vi "Scan Module.vi"(0 "#B scans":u32=1300, 1 "Channel":u32(ring)=1 items=["A"=1, "B"=2, "A + B"=3, "C"=4, "A + C"=5, "A + B"=6, "D"=8, "A + D"=9, "B + D"=10, "C + D"=12, "A + B + C + D"=15], 11 "Error In":errorcluster, 12 "Start Acquire?":bool) -> (3 "XY Graph":cluster{"X":dbl, "Y":dbl}[](graph), 4 "Finished?":bool, 6 "Ready for next C-scan?":bool, 8 "Current Position":cluster{"X":dbl, "Y":dbl}, 10 "Current state":T1, 15 "Error Out":errorcluster)   [LabVIEW 2018]
uses:
  Controls/Go Scan Actions.ctl
  Controls/FGV Actions.ctl
  Hardware Mfg/Thorlabs Translation Stages/Controls/Motion Translation Module Control.ctl
  Controls/Set Get Controls.ctl
  Hardware Mfg/Thorlabs Translation Stages/Controls/Translation Stage Cluster.ctl
  Controls/Translation Stage Types.ctl
  Hardware Mfg/AlazarTech SDK/Controls/Alazar Engine Actions.ctl
panel:
  out "Waveform Chart":dbl(graph)
  in  "No Slice?":bool
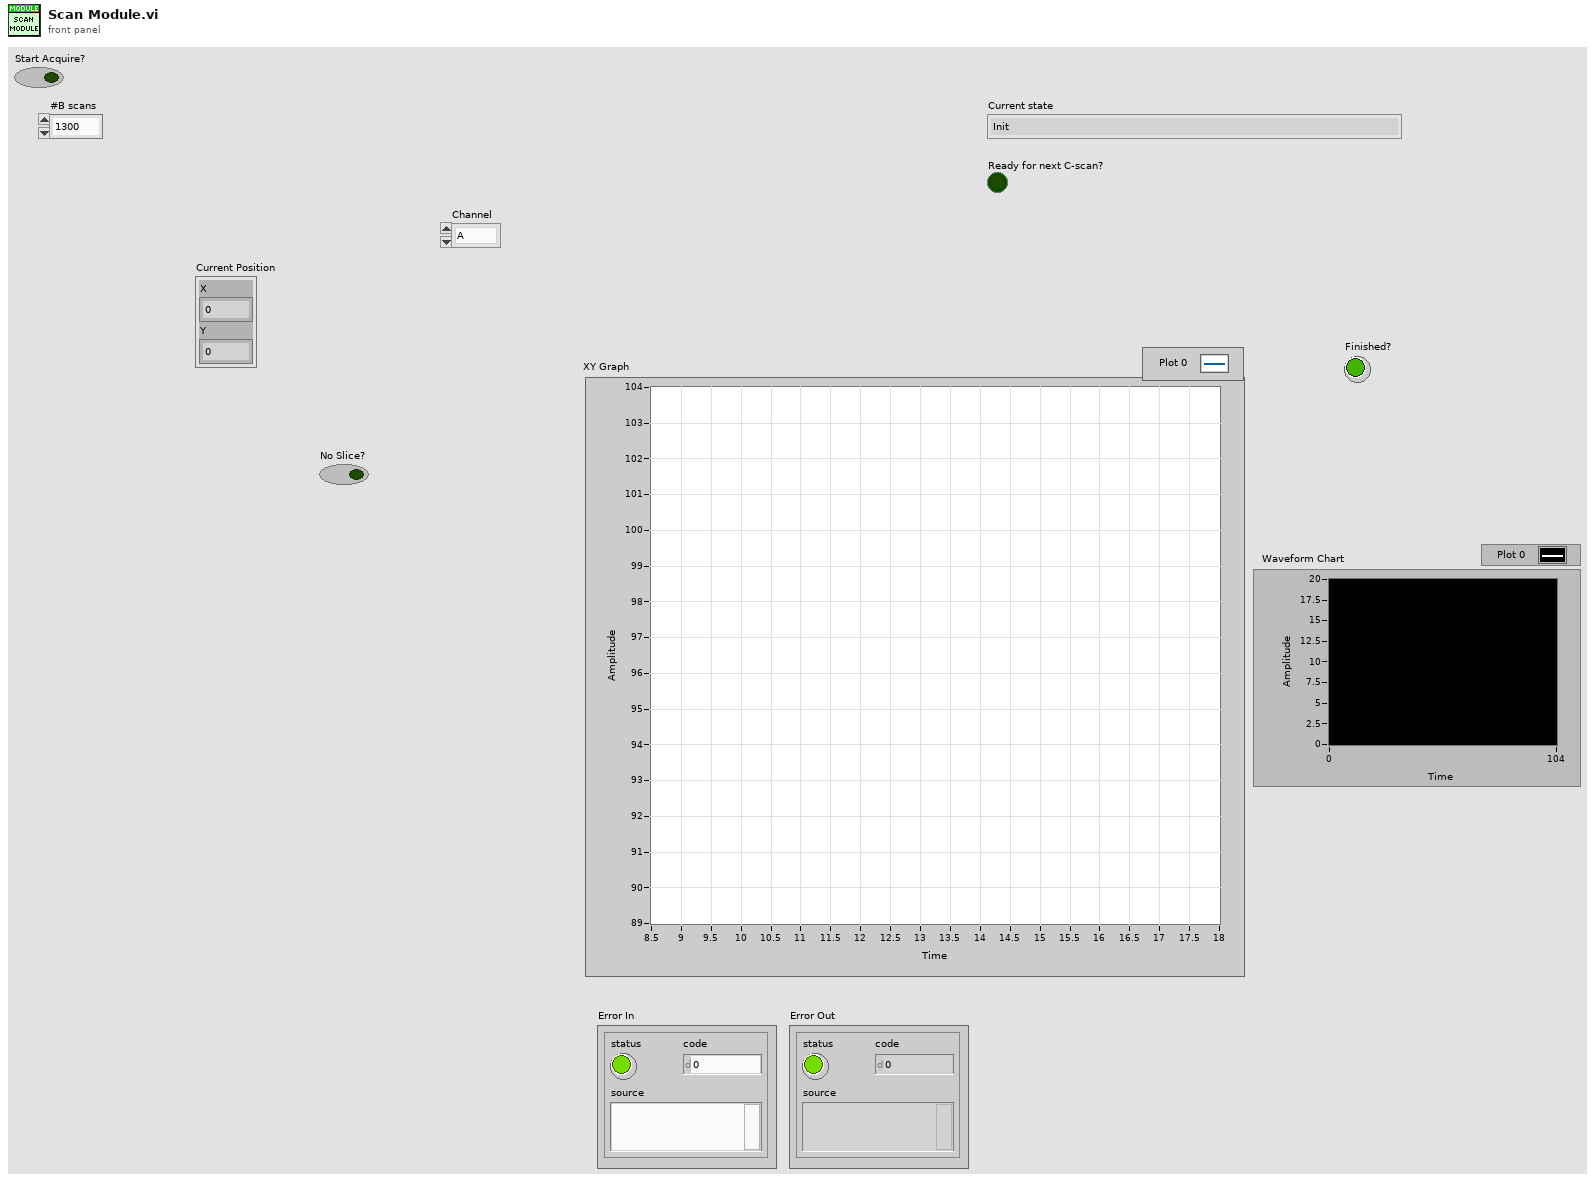
[diagram p1: front panel]
types:
  T1 = typedef "Go Scan Actions.ctl" = enum16{"Init", "Ready for acquire", "Init Scan Head", "Init Table Stage", "Init Vibratome", "Generate Mosaic", "Export info", "Go Image Home", "Go Mosaic", "Acquire Image", "Go Vibratome", "Slice", "Finished"}
  T2 = typedef "FGV Actions.ctl" = enum16{"Init", "Set", "Get", "Clear"}
  T3 = typedef "Translation Stage Cluster.ctl" = cluster{"Position":dbl, "Is.Enabled?":bool, "Is.Connected?":bool, "Device SN":string, "AccelerationMaximum":dbl, "VelocityMaximum":dbl, "Acceleration":dbl, "Velocity":dbl, "waitTimeout (ms)":i32, "Model":T4, "Is.Homed?":bool}
  T4 = typedef "Translation Stage Types.ctl" = enum16{"None", "Thorlabs LTS", "Thorlabs MLJ"}
  T5 = typedef "Set Get Controls.ctl" = enum16{"Set", "Get"}
  T6 = typedef "Motion Translation Module Control.ctl" = enum16{"Init", "Home", "Status", "Velocity/Accel", "Position", "Jog", "Stop", "Uninit", "Enable", "Disable"}
  T7 = enum16{"Configure channels", "Write Scan Pattern", "Start Galvo Task", "Is Task Done?", "Stop Galvo", "Uninit", "Init: Calc scan pattern"}
  T8 = typedef "Alazar Engine Actions.ctl" = enum16{"Init", "Config Clock", "Config Ch", "Config Trig", "Config Non-FFT Acq.", "Non-FFT Acquire", "Load background from Non-FFT buffer", "enable background subtrac", "disable background subtrac", "load background from file", "load background from elsewhere", "start acquire", "background subtraction", "Config Acq.", "Acquire", "UnInit"}
  T9 = typedef "Hardware control.ctl" = enum16{"PSOCT", "Thorlabs OCT"}
  T10 = typedef "ScanType.ctl" = enum16{"Single Frame", "Continuous Frame", "ROI Line", "Vibratome", "Mosaic", "Mosaic + Slice"}
  T11 = typedef "System Parameters.ctl" = cluster{"Optical Parameters":T12, "Vibratome":T13, "Table Stages":T14, "Imaging Parameter":T15, "Galvo HW Parameters":cluster{"Analog Out Channel":tag, "Min Voltage":dbl, "Max Voltage":dbl, "Pixel Clock Source":tag, "Sample Rate":dbl, "Line Clock Out Ch":tag}, "Alazar parameters":T17, "Mosaic Paramter":cluster{"X Axis":cluster{"Start [mm]":dbl, "Steps [pts]":u16, "End [mm]":dbl}, "Y Axis":cluster{"Start [mm]":dbl, "Steps [pts]":u16, "End [mm]":dbl}, "Scan Pattern":enum16{"Uni-directional", "Bi-Directional", "Spiral Out", "Spiral In"}, "Overlap Options":cluster{"Overlap Type":enum16{"No Overlap", "X Only", "Y Only", "X and Y"}, "Percent Overlap":u8, "Justify":enum16{"Start", "Center", "End"}}}}
  T12 = typedef "Optical Parameters.ctl" = cluster{"Obj. Focal Length [mm]":dbl, "Scan Lens EFL[mm]":dbl, "Tube Lens EFL[mm]":dbl, "Galvo V Range (+/-)":dbl, "Galvo Max Half Angle [Deg]":dbl, "Max Galvo Range[%]":dbl}
  T13 = typedef "Vibratome Parameters.ctl" = cluster{"Z Bottom [mm]":dbl, "Pre Cut Dwell [s]":dbl, "Blade Frequency [RPM]":u16, "Slice Speed [mm/s]":dbl, "Post Cut Dwell [s]":dbl, "Ramp Time [s]":dbl, "Start X [mm]":dbl, "Start Y [mm]":dbl, "Slice Length [mm]":dbl, "Slice Axis":enum16{"X Axis", "Y Axis", "Z Axis"}, "Controller VISA Ref":refnum<visa-resource-name>}
  T14 = typedef "Translation Stage Parameters.ctl" = cluster{"X Stage":T3, "Y Stage":T3, "Z Stage":T3}
  T15 = typedef "Imaging Parameters.ctl" = cluster{"Raster Scan Direction":T16, "Pixel Dwell Time [Clock Cycles]":u16, "Flyback Time [Clock Cycles]":u16, "XY Center [um]":cluster{"X":dbl, "Y":dbl}, "Pixel Step Size [um]":dbl, "XY Image Size":enum16{"32 x 32", "64 x 64", "128 x 128", "256 x 256", "512 x 512", "1024 x 1024", "2048 x 2048"}, "Custom":bool, "Custom Size":cluster{"X":u16, "Y":u16}, "Line Averages":u8}
  T16 = typedef "Scan Direction.ctl" = enum16{"Uni Directional", "Bi Directional", "None"}
  T17 = typedef "Alazar parameters.ctl" = cluster{"Trigger Settings":cluster{"General Trigger Settings":T18, "Trigger Engine 1":T19, "Trigger Engine 2":T19}, "Capture Clock":T20, "Device ID":T21, "Ch A Input Control":T22, "Ch B Input Control":T22, "Acq Settings":T23}
  T18 = typedef "General Trigger Settings.ctl" = cluster{"Trigger Operation":u32, "Coupling ID":u32, "Range ID":u32, "Delay":u32, "Timeout Ticks":u32, "Mode":u32, "Parameter":u32}
  T19 = typedef "Trigger Engine Controls.ctl" = cluster{"Trigger Engine":u32, "Source":u32, "Slope":u32, "Level":u32}
  T20 = typedef "Clock Controls.ctl" = cluster{"Sample Rate":u32, "Decimation":u32, "Source":u32, "Edge":u32}
  T21 = typedef "Alazar Device ID.ctl" = cluster{"System ID":u32, "Board ID":u32}
  T22 = typedef "Channel Input Controls.ctl" = cluster{"Channel":u8, "Coupling":u32, "Range":u32, "Impedance":u32}
  T23 = typedef "Alazar Acquisition Settings.ctl" = cluster{"Window Type":u32, "Record Length":u32, "Footer":u32, "Offset":u32, "Records Per Buffer":u32, "Samples per record":u32, "Records Count (Records/Acq)":u32, "Output Format":u32}
  T24 = cluster{"X Axis":cluster{"Start [mm]":dbl, "Steps [pts]":u16, "End [mm]":dbl}, "Y Axis":cluster{"Start [mm]":dbl, "Steps [pts]":u16, "End [mm]":dbl}, "Scan Pattern":enum16{"Uni-directional", "Bi-Directional", "Spiral Out", "Spiral In"}, "Overlap Options":cluster{"Overlap Type":enum16{"No Overlap", "X Only", "Y Only", "X and Y"}, "Percent Overlap":u8, "Justify":enum16{"Start", "Center", "End"}}}
  T25 = cluster{"Start [mm]":dbl, "Steps [pts]":u16, "End [mm]":dbl}
  T26 = cluster{"Overlap Type":enum16{"No Overlap", "X Only", "Y Only", "X and Y"}, "Percent Overlap":u8, "Justify":enum16{"Start", "Center", "End"}}
  T27 = enum16{"Uni-directional", "Bi-Directional", "Spiral Out", "Spiral In"}
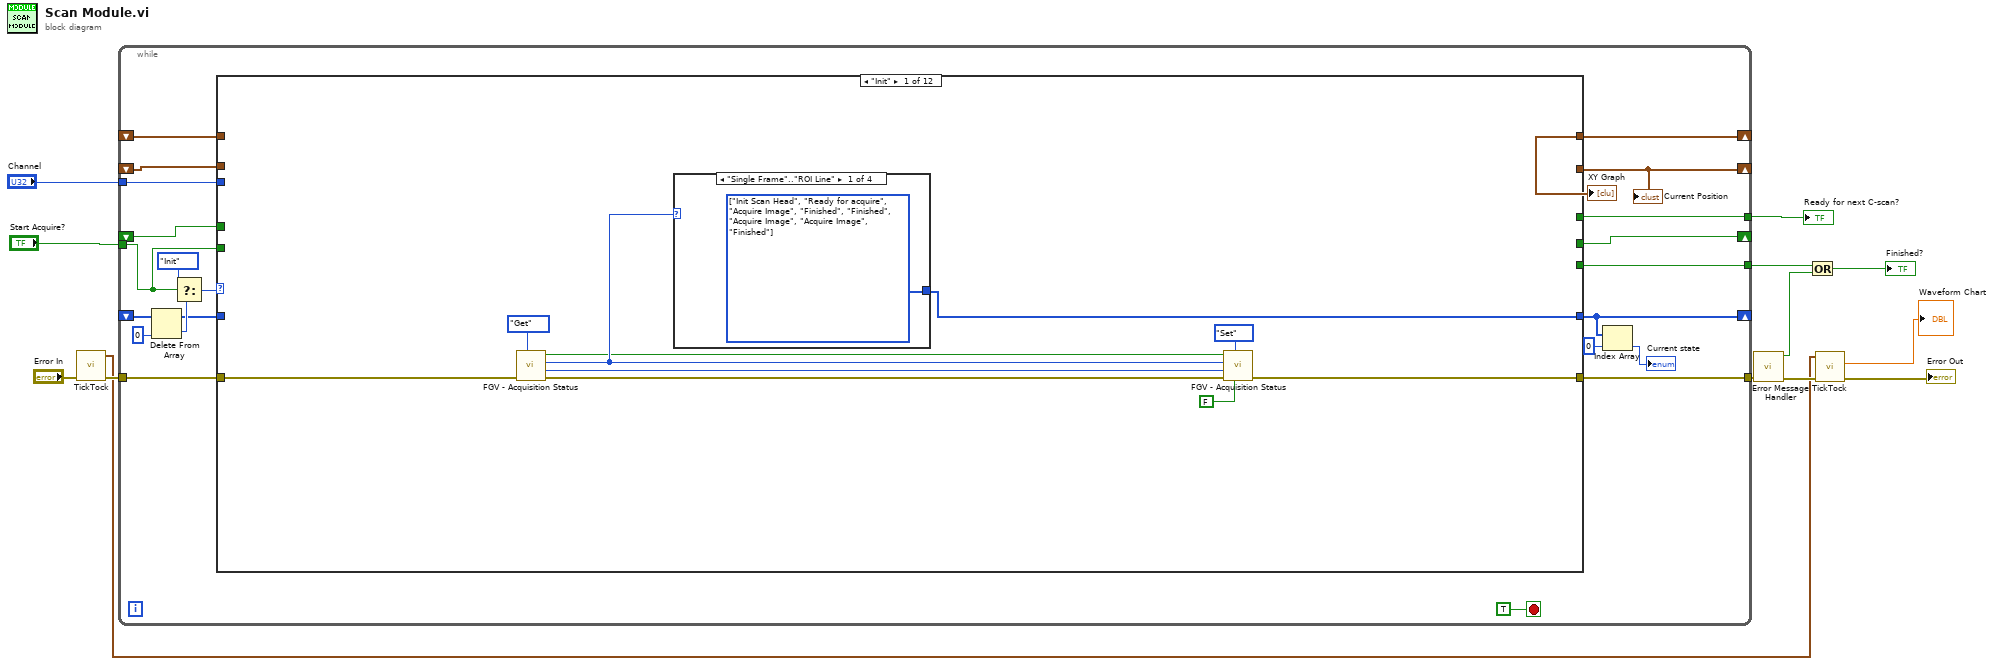
[diagram p0: block diagram]
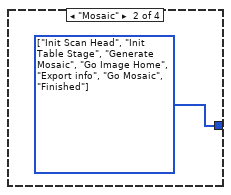
[diagram p2: hidden frame]
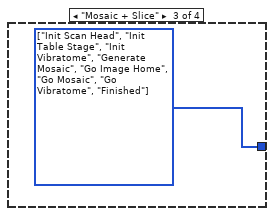
[diagram p3: hidden frame]
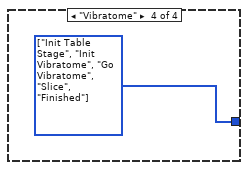
[diagram p4: hidden frame]
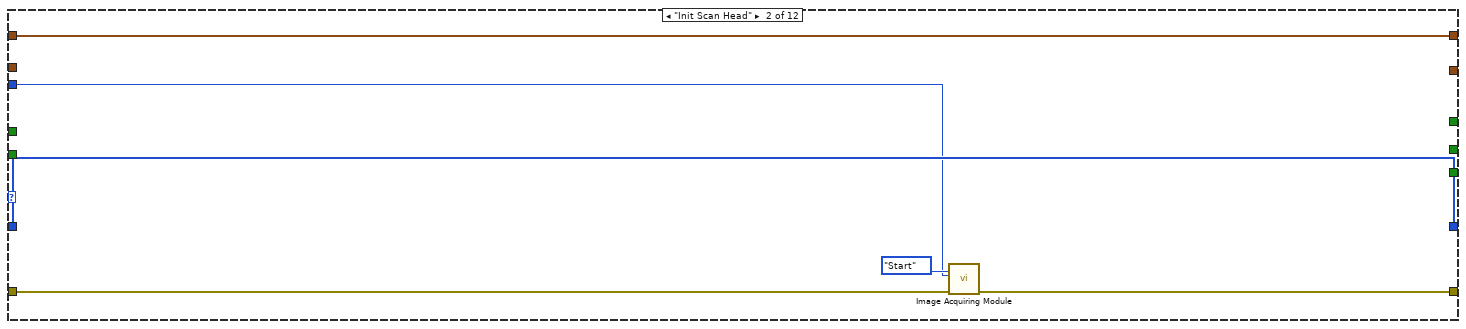
[diagram p5: hidden frame]
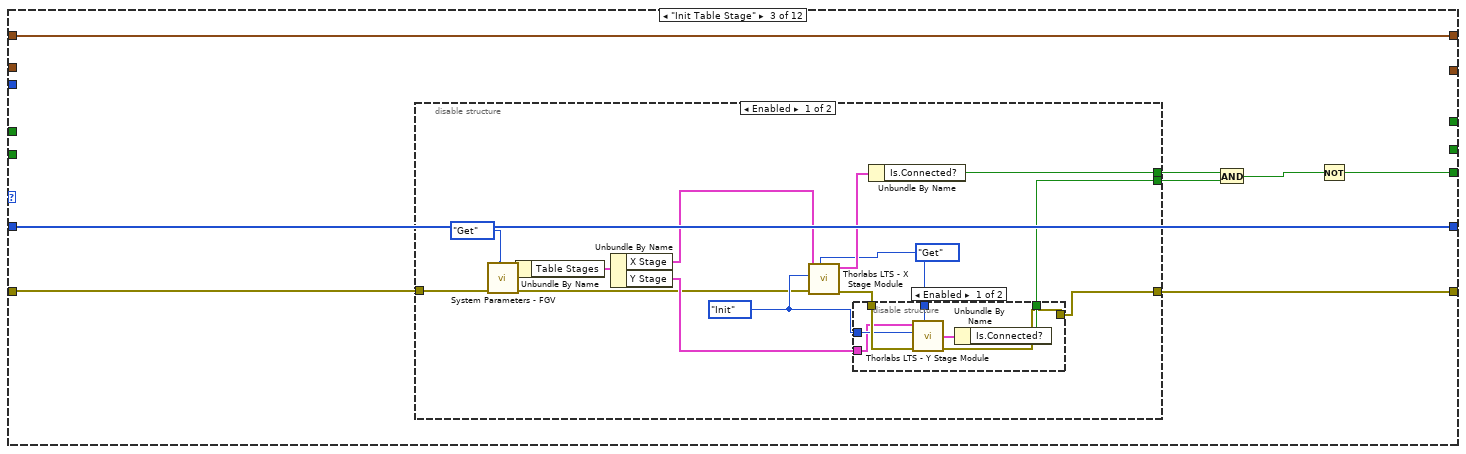
[diagram p6: hidden frame]
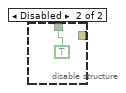
[diagram p7: hidden frame]
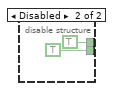
[diagram p8: hidden frame]
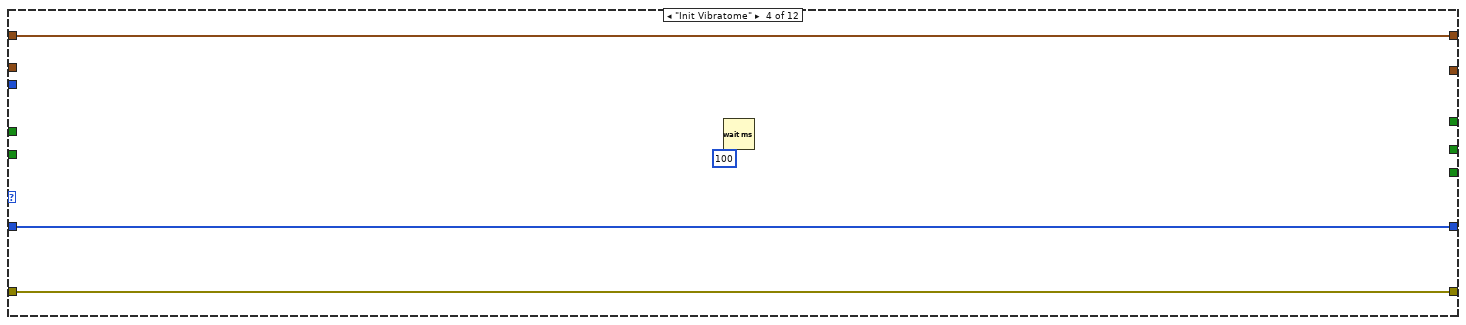
[diagram p9: hidden frame]
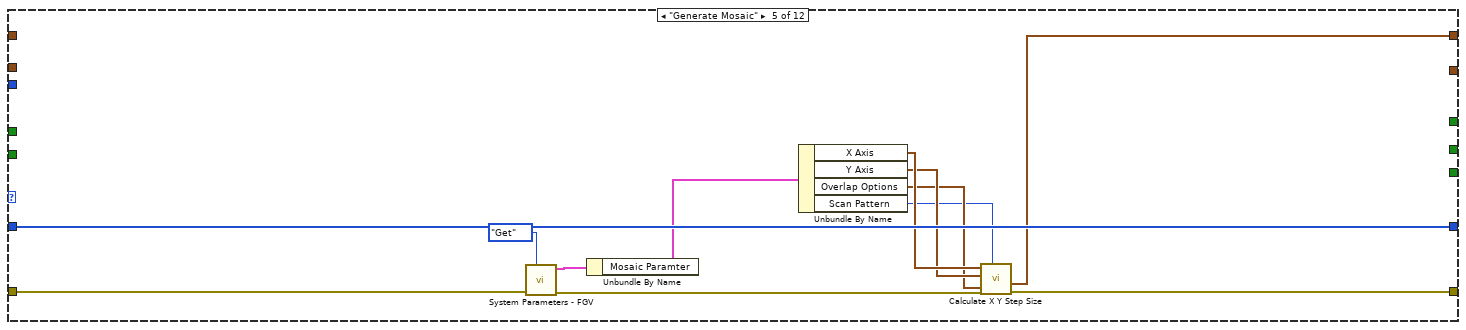
[diagram p10: hidden frame]
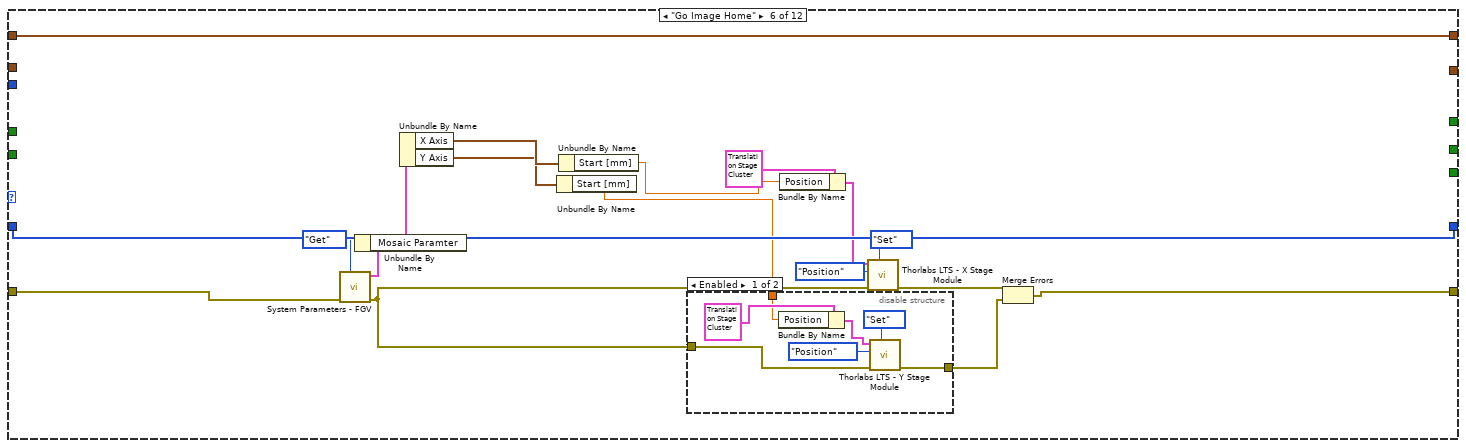
[diagram p11: hidden frame]
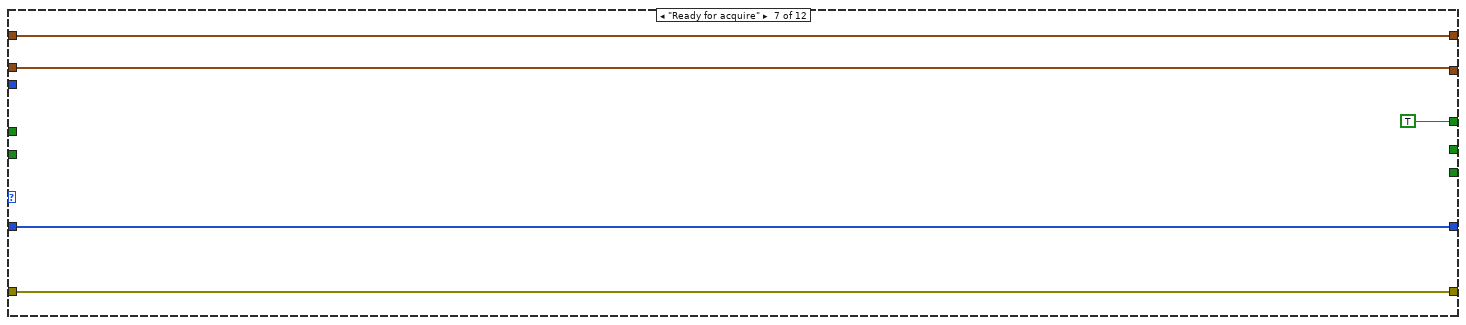
[diagram p13: hidden frame]
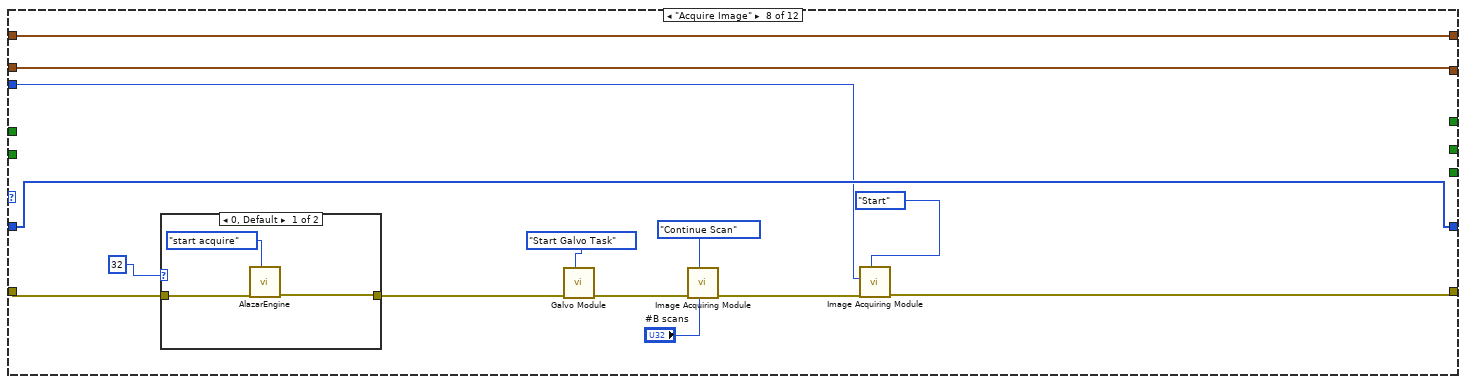
[diagram p14: hidden frame]
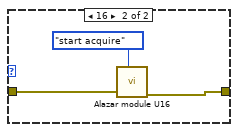
[diagram p15: hidden frame]
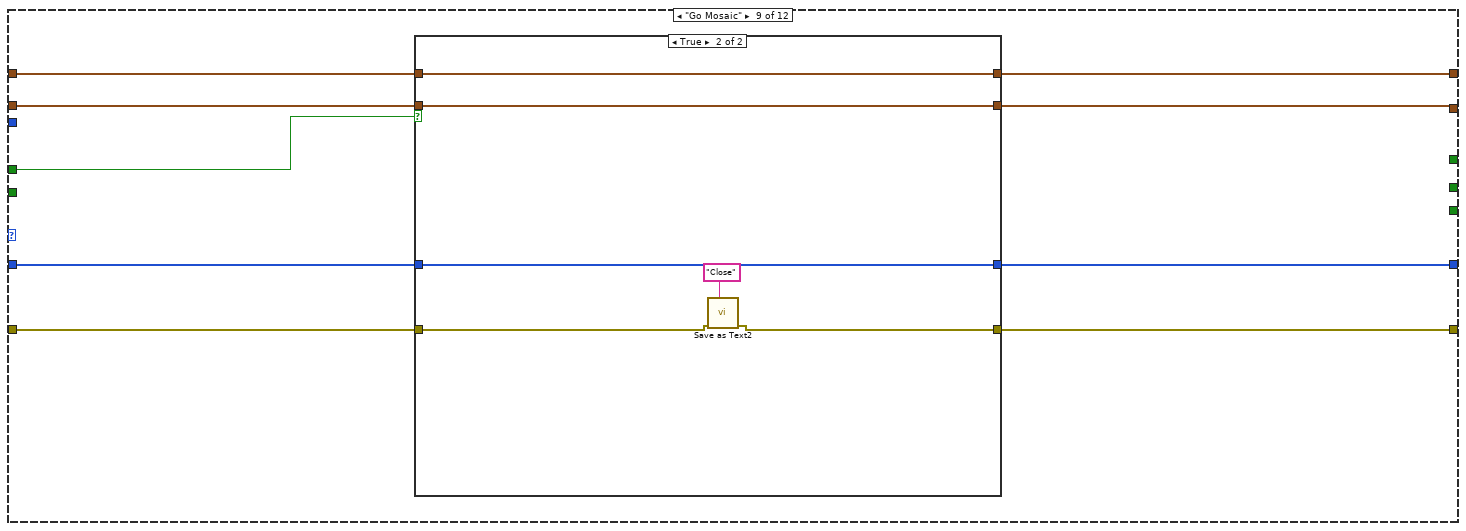
[diagram p16: hidden frame]
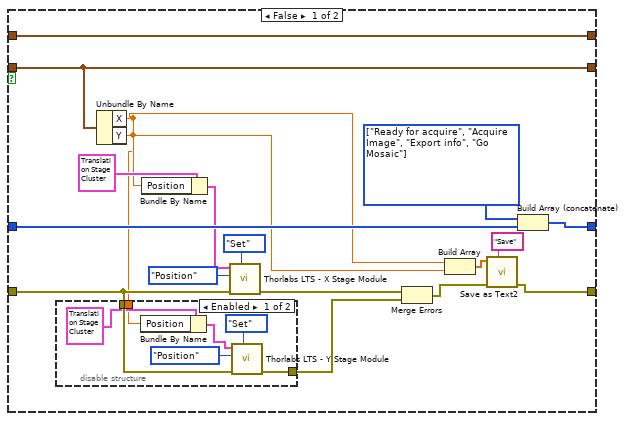
[diagram p17: hidden frame]
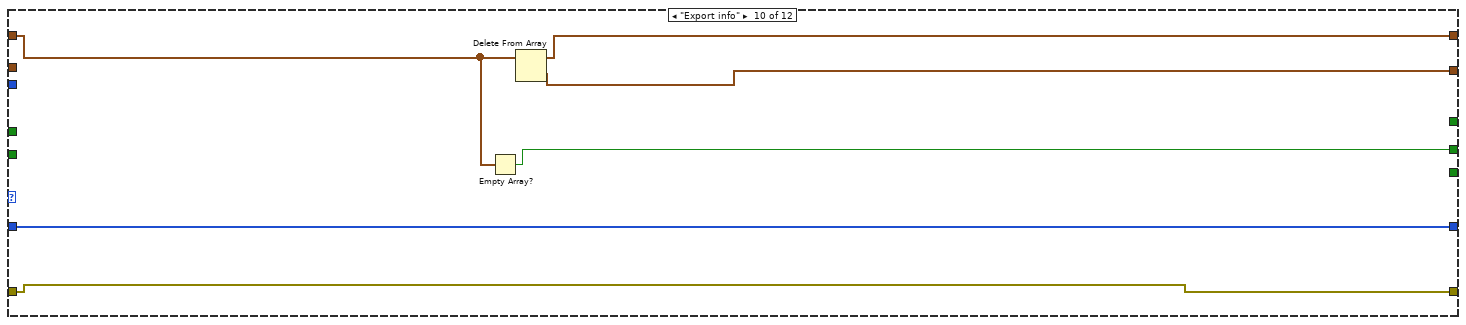
[diagram p19: hidden frame]
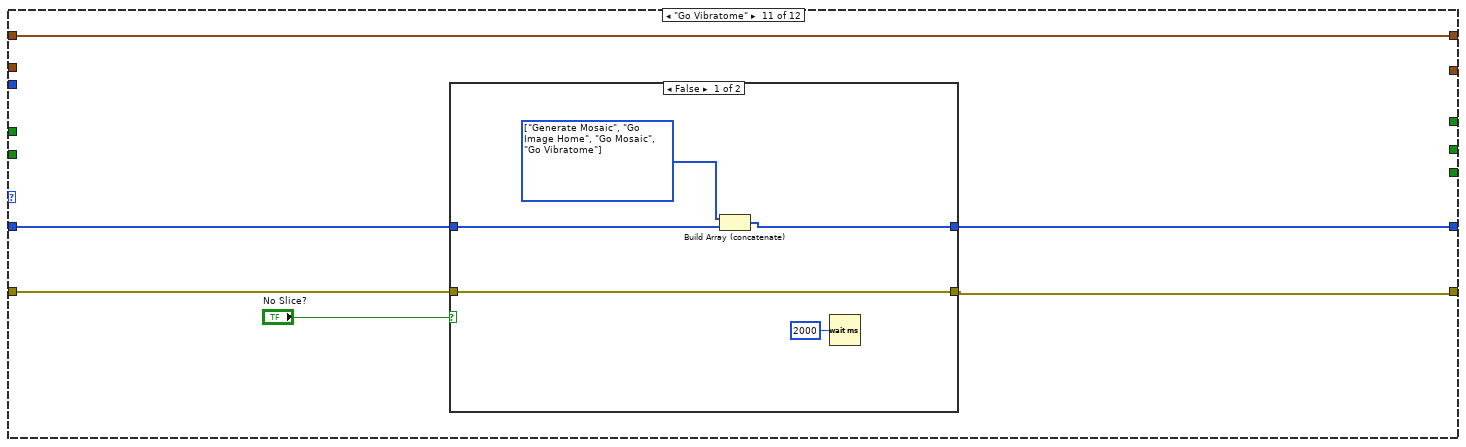
[diagram p20: hidden frame]
diagram:
  n1 = call "TickTock.vi"("Error In"="Error In") -> ("Error Out"=w7:errorcluster, "Current Time (Out)"=w5:timestamp)  [unwired: 8 in, 1 out]
  n2 = while {
    shift-right: [w16] -> _
    shift-left: _ -> [w33]
    tunnel: "Start Acquire?" -> [w23]
    shift-right: [w29] -> _
    shift-left: _ -> [w30]
    tunnel: [w28] -> w13
    tunnel: w7 -> [w26]
    tunnel: [w25] -> w12
    tunnel: [w22] -> w2
    tunnel: "Channel" -> [w21]
    shift-right: [w14] -> _
    shift-left: _ -> [w18]
    shift-right: [w20] -> _
    shift-left: _ -> [w19]
    stop <- TRUE stop-if-true
    n3 = Delete From Array(array=w33, index=0) -> (deleted portion=w32:T1, array with subset deleted=w31:T1[])  [unwired: 1 in]
    n4 = Select(t=Go_Scan_Actions."Init", s=w23, f=w32) -> (s? t:f=w24:T1)
    n5 = case shown="\"Init\"" w24 {
      tunnel: [w43 w54 w62 w90 w103 w121 w130 w146 w157 w196 w200 _] -> w16
      tunnel: w31 -> [_ w54 w62 w90 w103 w121 w130 w146 w160 w196 w203 _]
      tunnel: [_ w55 w63 w91 w102 w120 w132 w147 w162 w199 w205 _] -> w29
      tunnel: w30 -> [_ w55 w63 w91 _ w120 w132 w147 w161 w198 w205 _]
      tunnel: [_ _ w60 _ _ _ _ _ _ _ _ TRUE] -> w28
      tunnel: w26 -> [w44 w50 w57 w88 w93 w106 w133 w142 w159 w194 w202 w222]
      tunnel: [w41 w52 w56 w88 w92 w104 w133 w138 w158 w194 w201 w214] -> w25
      tunnel: w23 -> [_ _ _ _ _ _ _ _ _ _ _ _]
      tunnel: [_ _ _ _ _ _ TRUE _ _ _ _ _] -> w22
      tunnel: w21 -> [_ w51 _ _ _ _ _ w139 _ _ _ _]
      tunnel: [_ _ _ _ _ _ w129 w134 w154 w195 _ _] -> w14
      tunnel: [_ _ _ _ _ _ _ _ _ w197 _ _] -> w20
      tunnel: w19 -> [_ _ _ _ _ _ _ _ w156 _ _ _]
      tunnel: w18 -> [_ _ _ _ _ _ w129 w134 w155 _ _ _]
      frame "Init" {
        n6 = call "FGV - Acquisition Status.vi"("Actions"=FGV_Actions."Get", "Error In"=w44) -> ("Error Out"=w42:errorcluster, "Hardware out"=w39:T9, "Scan Type [Out]"=w38:T10, "Level Status Out"=w37:bool)  [unwired: 5 in, 1 out]
        n7 = case shown="\"Single Frame\"..\"ROI Line\"" w38 {
          tunnel: [w46 w47 w48 w49] -> w43
          frame "Single Frame".."ROI Line" {
            w46 = T1[] [enum."Init Scan Head", enum."Ready for acquire", enum."Acquire Image", enum."Finished", enum."Finished", enum."Acquire Image", enum."Acquire Image", enum."Finished"] items=["Init", "Ready for acquire", "Init Scan Head", "Init Table Stage", "Init Vibratome", "Generate Mosaic", "Export info", "Go Image Home", "Go Mosaic", "Acquire Image", "Go Vibratome", "Slice", "Finished"]
          }
          frame "Mosaic" {
            w47 = T1[] [enum."Init Scan Head", enum."Init Table Stage", enum."Generate Mosaic", enum."Go Image Home", enum."Export info", enum."Go Mosaic", enum."Finished"] items=["Init", "Ready for acquire", "Init Scan Head", "Init Table Stage", "Init Vibratome", "Generate Mosaic", "Export info", "Go Image Home", "Go Mosaic", "Acquire Image", "Go Vibratome", "Slice", "Finished"]
          }
          frame "Mosaic + Slice" {
            w48 = T1[] [enum."Init Scan Head", enum."Init Table Stage", enum."Init Vibratome", enum."Generate Mosaic", enum."Go Image Home", enum."Go Mosaic", enum."Go Vibratome", enum."Finished"] items=["Init", "Ready for acquire", "Init Scan Head", "Init Table Stage", "Init Vibratome", "Generate Mosaic", "Export info", "Go Image Home", "Go Mosaic", "Acquire Image", "Go Vibratome", "Slice", "Finished"]
          }
          frame "Vibratome" {
            w49 = T1[] [enum."Init Table Stage", enum."Init Vibratome", enum."Go Vibratome", enum."Slice", enum."Finished"] items=["Init", "Ready for acquire", "Init Scan Head", "Init Table Stage", "Init Vibratome", "Generate Mosaic", "Export info", "Go Image Home", "Go Mosaic", "Acquire Image", "Go Vibratome", "Slice", "Finished"]
          }
        }
        n8 = call "FGV - Acquisition Status.vi"("Edge Status In"=FALSE, "Actions"=FGV_Actions."Set", "Error In"=w42, "Hardware in"=w39, "Scan Type [In]"=w38, "Level Status In"=w37) -> ("Error Out"=w41:errorcluster)  [unwired: 1 in, 4 out]
      }
      frame "Init Scan Head" {
        n9 = call "Image Acquiring Module.vi"("Scan Status in"=enum16{"Start", "Continue Scan", "Finish Scan"}."Start", "Error in"=w50, "Channel"=w51) -> ("Error Out"=w52:errorcluster)  [unwired: 8 in]
      }
      frame "Init Table Stage" {
        n10 = disable-structure shown="Enabled" {
          disable-tunnel: [w75 TRUE ("Is.Connected?")] -> w61
          disable-tunnel: [w73 TRUE ("Is.Connected?")] -> w58
          disable-tunnel: w57 -> [w66 _]
          disable-tunnel: [w64 _] -> w56
          frame Enabled {
            w72 = Set_Get_Controls."Get" ("Set/Get")
            w74 = Motion_Translation_Module_Control."Init" ("Action")
            n11 = call "System Parameters - FGV.vi"("Actions"=FGV_Actions."Get", "Error In"=w66) -> ("Error Out"=w65:errorcluster, "System Parameters"=w70:T11)  [unwired: 8 in]
            n12 = Unbundle By Name(w70) -> ("Table Stages"=w69:T14)
            n13 = Unbundle By Name(w69) -> ("X Stage"=w68:T3, "Y Stage"=w67:T3)
            n14 = call "Thorlabs LTS - X Stage Module.vi"("Set/Get"=w72, "Error In"=w65, "Action"=w74, "Cluster In"=w68) -> ("Error Out"=w77:errorcluster, "Cluster Out"=w76:T3)  [unwired: 6 in]
            n15 = disable-structure shown="Enabled" {
              disable-tunnel: w77 -> [w84 _]
              disable-tunnel: w74 -> [w83 _]
              disable-tunnel: [w81 TRUE] -> w73
              disable-tunnel: w72 -> [w80 _]
              disable-tunnel: w67 -> [w79 _]
              disable-tunnel: [w78 _] -> w64
              frame Enabled {
                n16 = call "Thorlabs LTS - Y Stage Module.vi"("Set/Get"=w80, "Error In"=w84, "Action"=w83, "Cluster In"=w79) -> ("Error Out"=w78:errorcluster, "Cluster Out"=w82:T3)  [unwired: 6 in]
                n17 = Unbundle By Name(w82) -> ("Is.Connected?"=w81:bool)
              }
              frame Disabled {
              }
            }
            n18 = Unbundle By Name(w76) -> ("Is.Connected?"=w75:bool)
          }
          frame Disabled {
          }
        }
        n19 = And(x=w61, y=w58) -> (x .and. y?=w59:bool)
        n20 = Not(x=w59) -> (.not. x?=w60:bool)
      }
      frame "Init Vibratome" {
        n21 = Wait (ms)(milliseconds to wait=u32 100) -> ()  [unwired: 1 out]
      }
      frame "Generate Mosaic" {
        n22 = call "System Parameters - FGV.vi"("Actions"=FGV_Actions."Get", "Error In"=w93) -> ("Error Out"=w97:errorcluster, "System Parameters"=w95:T11)  [unwired: 8 in]
        n23 = Unbundle By Name(w95) -> ("Mosaic Paramter"=w94:T24)
        n24 = Unbundle By Name(w94) -> ("X Axis"=w101:T25, "Y Axis"=w100:T25, "Overlap Options"=w99:T26, "Scan Pattern"=w98:T27)
        n25 = call "Calculate X Y Step Size.vi"("Overlap Options"=w99, "Scan Pattern"=w98, "Error In"=w97, "Y Axis"=w100, "X Axis"=w101) -> ("Error Out"=w92:errorcluster, "Array"=w102:cluster{"X":dbl, "Y":dbl}[])  [unwired: 3 in, 2 out]
      }
      frame "Go Image Home" {
        n26 = call "System Parameters - FGV.vi"("Actions"=FGV_Actions."Get", "Error In"=w106) -> ("Error Out"=w105:errorcluster, "System Parameters"=w112:T11)  [unwired: 8 in]
        n27 = Unbundle By Name(w112) -> ("Mosaic Paramter"=w111:T24)
        n28 = Unbundle By Name(w111) -> ("X Axis"=w110:T25, "Y Axis"=w109:T25)
        n29 = Unbundle By Name(w109) -> ("Start [mm]"=w107:dbl)
        n30 = Unbundle By Name(w110) -> ("Start [mm]"=w108:dbl)
        n31 = disable-structure shown="Enabled" {
          disable-tunnel: [w124 _] -> w114
          disable-tunnel: w107 -> [w123 _]
          disable-tunnel: w105 -> [w122 _]
          frame Enabled {
            n32 = Bundle By Name(cluster=T3 {"Position"=0.0, "Is.Enabled?"=FALSE, "Is.Connected?"=FALSE, "Device SN"="45876539", "AccelerationMaximum"=0.0, "VelocityMaximum"=0.0, "Acceleration"=0.0, "Velocity"=0.0, "waitTimeout (ms)"=10000, "Model"=enum."None", "Is.Homed?"=FALSE} ("Cluster In"), "Position"=w123) -> (w125:T3)
            n33 = call "Thorlabs LTS - Y Stage Module.vi"("Set/Get"=Set_Get_Controls."Set", "Error In"=w122, "Action"=Motion_Translation_Module_Control."Position", "Cluster In"=w125) -> ("Error Out"=w124:errorcluster)  [unwired: 6 in, 1 out]
          }
          frame Disabled {
          }
        }
        n34 = Bundle By Name(cluster=T3 {"Position"=0.0, "Is.Enabled?"=FALSE, "Is.Connected?"=FALSE, "Device SN"="45876539", "AccelerationMaximum"=0.0, "VelocityMaximum"=0.0, "Acceleration"=0.0, "Velocity"=0.0, "waitTimeout (ms)"=10000, "Model"=enum."None", "Is.Homed?"=FALSE} ("Cluster In"), "Position"=w108) -> (w115:T3)
        n35 = call "Thorlabs LTS - X Stage Module.vi"("Set/Get"=Set_Get_Controls."Set", "Error In"=w105, "Action"=Motion_Translation_Module_Control."Position", "Cluster In"=w115) -> ("Error Out"=w118:errorcluster)  [unwired: 6 in, 1 out]
        n36 = Merge Errors(w118, w114) -> (w104:errorcluster)
      }
      frame "Ready for acquire" {
      }
      frame "Acquire Image" {
        n37 = case shown="0, Default" 32 {
          tunnel: w142 -> [w150 w153]
          tunnel: [w149 w152] -> w137
          frame 0, Default {
            n38 = call "AlazarEngine.vi"("Action"=Alazar_Engine_Actions."start acquire", "error in (no error)"=w150) -> ("error out"=w149:errorcluster)  [unwired: 7 in, 2 out]
          }
          frame 16 {
            n39 = call "Alazar module U16.vi"("Action"=Alazar_Engine_Actions."start acquire", "error in (no error)"=w153) -> ("error out"=w152:errorcluster)  [unwired: 7 in, 2 out]
          }
        }
        n40 = call "Galvo Module.vi"("Action"=T7."Start Galvo Task", "error in (no error)"=w137) -> ("error out"=w143:errorcluster)  [unwired: 8 in, 1 out]
        n41 = call "Image Acquiring Module.vi"("#B scans"="#B scans", "Scan Status in"=enum16{"Start", "Continue Scan", "Finish Scan"}."Continue Scan", "Error in"=w143) -> ("Error Out"=w141:errorcluster)  [unwired: 8 in]
        n42 = call "Image Acquiring Module.vi"("Scan Status in"=enum16{"Start", "Continue Scan", "Finish Scan"}."Start", "Error in"=w141, "Channel"=w139) -> ("Error Out"=w138:errorcluster)  [unwired: 8 in]
      }
      frame "Go Mosaic" {
        n43 = case shown="True" w156 {
          tunnel: [w170 w193] -> w162
          tunnel: w161 -> [w170 w193]
          tunnel: w160 -> [w180 w192]
          tunnel: [w179 w192] -> w157
          tunnel: w159 -> [w172 w189]
          tunnel: [w166 w188] -> w158
          tunnel: w155 -> [w163 w191]
          tunnel: [w163 w191] -> w154
          frame False {
            w178 = T1[] [enum."Ready for acquire", enum."Acquire Image", enum."Export info", enum."Go Mosaic"] items=["Init", "Ready for acquire", "Init Scan Head", "Init Table Stage", "Init Vibratome", "Generate Mosaic", "Export info", "Go Image Home", "Go Mosaic", "Acquire Image", "Go Vibratome", "Slice", "Finished"]
            n44 = Unbundle By Name(w163) -> ("X"=w165:dbl, "Y"=w164:dbl)
            n45 = disable-structure shown="Enabled" {
              disable-tunnel: w172 -> [w185 _]
              disable-tunnel: w164 -> [w183 _]
              disable-tunnel: [w181 _] -> w171
              frame Enabled {
                n46 = Bundle By Name(cluster=T3 {"Position"=0.0, "Is.Enabled?"=FALSE, "Is.Connected?"=FALSE, "Device SN"="45876539", "AccelerationMaximum"=0.0, "VelocityMaximum"=0.0, "Acceleration"=0.0, "Velocity"=0.0, "waitTimeout (ms)"=10000, "Model"=enum."None", "Is.Homed?"=FALSE} ("Cluster In"), "Position"=w183) -> (w182:T3)
                n47 = call "Thorlabs LTS - Y Stage Module.vi"("Set/Get"=Set_Get_Controls."Set", "Error In"=w185, "Action"=Motion_Translation_Module_Control."Position", "Cluster In"=w182) -> ("Error Out"=w181:errorcluster)  [unwired: 6 in, 1 out]
              }
              frame Disabled {
              }
            }
            n48 = Bundle By Name(cluster=T3 {"Position"=0.0, "Is.Enabled?"=FALSE, "Is.Connected?"=FALSE, "Device SN"="45876539", "AccelerationMaximum"=0.0, "VelocityMaximum"=0.0, "Acceleration"=0.0, "Velocity"=0.0, "waitTimeout (ms)"=10000, "Model"=enum."None", "Is.Homed?"=FALSE} ("Cluster In"), "Position"=w165) -> (w173:T3)
            n49 = call "Thorlabs LTS - X Stage Module.vi"("Set/Get"=Set_Get_Controls."Set", "Error In"=w172, "Action"=Motion_Translation_Module_Control."Position", "Cluster In"=w173) -> ("Error Out"=w176:errorcluster)  [unwired: 6 in, 1 out]
            n50 = Merge Errors(w176, w171) -> (w167:errorcluster)
            n51 = Build Array(w165, w164) -> (w169:dbl[])
            n52 = call "Save as Text2.vi"("action"="Save", "error in"=w167, "data in"=w169) -> ("error out"=w166:errorcluster)  [unwired: 8 in]
            n53 = Build Array (concatenate)(w178, w180) -> (w179:T1[])
          }
          frame True {
            n54 = call "Save as Text2.vi"("action"="Close", "error in"=w189) -> ("error out"=w188:errorcluster)  [unwired: 9 in]
          }
        }
      }
      frame "Export info" {
        n55 = Empty Array?(array=w198) -> (empty?=w197:bool)
        n56 = Delete From Array(array=w198) -> (deleted portion=w195:cluster{"X":dbl, "Y":dbl}, array with subset deleted=w199:cluster{"X":dbl, "Y":dbl}[])  [unwired: 2 in]
      }
      frame "Go Vibratome" {
        n57 = case shown="False" "No Slice?" {
          tunnel: w203 -> [w210 w212]
          tunnel: [w209 w212] -> w200
          tunnel: w202 -> [w206 w211]
          tunnel: [w206 w211] -> w201
          frame False {
            w208 = T1[] [enum."Generate Mosaic", enum."Go Image Home", enum."Go Mosaic", enum."Go Vibratome"] items=["Init", "Ready for acquire", "Init Scan Head", "Init Table Stage", "Init Vibratome", "Generate Mosaic", "Export info", "Go Image Home", "Go Mosaic", "Acquire Image", "Go Vibratome", "Slice", "Finished"]
            n58 = Build Array (concatenate)(w208, w210) -> (w209:T1[])
            n59 = Wait (ms)(milliseconds to wait=u32 2000) -> ()  [unwired: 1 out]
          }
          frame True {
          }
        }
      }
      frame "Finished", Default {
        n60 = call "Image Acquiring Module.vi"("Scan Status in"=enum16{"Start", "Continue Scan", "Finish Scan"}."Finish Scan", "Error in"=w222) -> ("Error Out"=w220:errorcluster)  [unwired: 9 in]
        n61 = call "FGV - Acquisition Status.vi"("Actions"=FGV_Actions."Get", "Error In"=w220) -> ("Error Out"=w221:errorcluster, "Hardware out"=w215:T9, "Scan Type [Out]"=w217:T10, "Edge Status Out"=w213:bool)  [unwired: 5 in, 1 out]
        n62 = call "FGV - Acquisition Status.vi"("Edge Status In"=w213, "Actions"=FGV_Actions."Set", "Error In"=w221, "Hardware in"=w215, "Scan Type [In]"=w217, "Level Status In"=FALSE ("Status In")) -> ("Error Out"=w214:errorcluster)  [unwired: 1 in, 4 out]
      }
    }
    "XY Graph" <- w29
    "Current Position" <- w14
    n63 = Index Array(array=w16, index=0) -> (element=→"Current state":T1)
  }
  "Ready for next C-scan?" <- w2
  n64 = call "Error Message Handler.vi"("Error In"=w12) -> ("Error Out"=w11:errorcluster, "T button?"=w9:bool)  [unwired: 9 in]
  n65 = Or(x=w13, y=w9) -> (x .or. y?=→"Finished?":bool)
  n66 = call "TickTock.vi"("Error In"=w11, "Current Time (In)"=w5) -> ("Error Out"=→"Error Out":errorcluster, "dt"=→"Waveform Chart":dbl)  [unwired: 7 in, 1 out]
